vi "TeslaSense Server mimic.vi"() -> ()   [LabVIEW 2019]
doc: "Demonstrates how to set up a basic TCP connection, send data to the specified port once a connection has been established, and terminate the connection once the data has been sent. This VI is designed to stop if the TCP connection is terminated. The data sent in this example is an array of random numbers."
panel:
  in  "Client Closed":string="The client VI closed the connection."
  in  "Stop":bool
  out "data read from client gui (timestamp, thresholds)":string
  out "Array of data read from GUI":dbl[](array[numeric])
  out "Timestamp":dbl
  out "appended array":dbl[](array[numeric])
  out "length":i32
  # "This program mimics the TeslaSense server so that the Client can be tested without the launchpad."
  # "1. Make sure bytes read on TeslaSense client is 82"
  # "2. Make sure TeslaSense client opens connection with 'localhost'"
  # "3. Start client first"
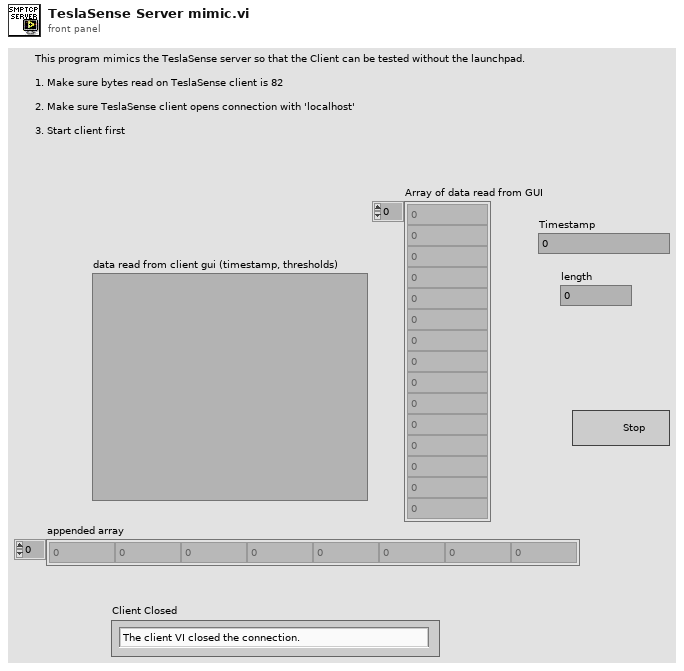
[diagram p1: front panel]
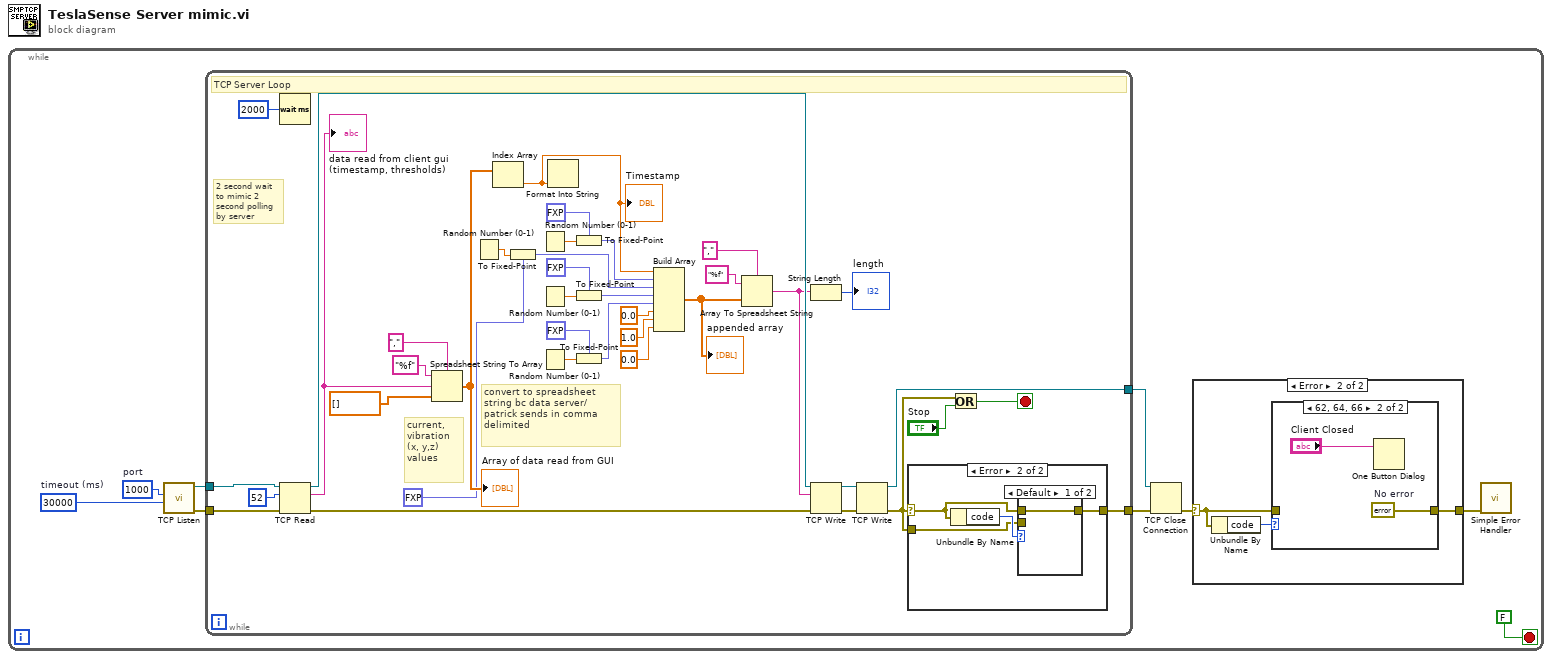
[diagram p0: block diagram]
diagram:
  n1 = while {
    stop <- FALSE stop-if-true
    w4 = u16 1000  # port
    w5 = 30000  # timeout (ms)
    n2 = call <vilib>:"TCP Listen.vi"("timeout ms (wait forever: -1)"=w5, "port"=w4) -> ("error out"=w6:errorcluster, "connection ID"=w7:refnum<k5>)  [unwired: 5 in, 3 out]
    n3 = while {
      tunnel: w7 -> [w38]
      tunnel: w6 -> [w37]
      tunnel: [w42] -> w3
      tunnel: [w41] -> w2
      stop <- w17 stop-if-true
      # "2 second wait to mimic 2 second polling by server"
      # "convert to spreadsheet string bc data server/patrick sends in comma delimited"
      # "current, vibration (x, y,z) values"
      # "TCP Server Loop"
      n4 = Wait (ms)(milliseconds to wait=u32 2000) -> ()  [unwired: 1 out]
      n5 = TCP Read(connection ID=w38, bytes to read=52, error in (no error)=w37) -> (connection ID out=w46:refnum<k5>, data out=w52:string, error out=w45:errorcluster)  [unwired: 2 in]
      "data read from client gui (timestamp, thresholds)" <- w52
      n6 = Spreadsheet String To Array(delimiter (Tab)=",", format string="%f", spreadsheet string=w52, array type (2D Dbl)=dbl[] []) -> (array=w51:dbl[])
      "Array of data read from GUI" <- w51
      n7 = Random Number (0-1)() -> (number: 0 to 1=w29:dbl)
      n8 = Index Array(array=w51) -> (element=w50:dbl)  [unwired: 1 in]
      "Timestamp" <- w50
      n9 = To Fixed-Point(fixed-point type=fxp<+/-,32,16> 10.0, number=w29) -> (fixed-point=w28:fxp<+/-,32,16>)
      n10 = Random Number (0-1)() -> (number: 0 to 1=w32:dbl)
      n11 = Random Number (0-1)() -> (number: 0 to 1=w25:dbl)
      n12 = Random Number (0-1)() -> (number: 0 to 1=w23:dbl)
      n13 = Format Into String(w50) -> ()  [unwired: 3 in, 2 out]
      n14 = To Fixed-Point(fixed-point type=fxp<+/-,32,16> 10.0, number=w32) -> (fixed-point=w31:fxp<+/-,32,16>)
      n15 = To Fixed-Point(fixed-point type=fxp<+/-,32,16> 10.0, number=w25) -> (fixed-point=w26:fxp<+/-,32,16>)
      n16 = To Fixed-Point(fixed-point type=fxp<+/-,32,16> 10.0, number=w23) -> (fixed-point=w22:fxp<+/-,32,16>)
      n17 = Build Array(w50, w31, w28, w26, w22, 0.0 ("element"), 1.0 ("element"), 0.0 ("element")) -> (w49:dbl[])
      "appended array" <- w49
      n18 = Array To Spreadsheet String(delimiter (Tab)=",", array=w49, 3:"%f" ("format string")) -> (spreadsheet string=w21:string)
      n19 = String Length(string=w21) -> (length=→"length":i32)
      n20 = TCP Write(connection ID=w46, data in=w21, error in (no error)=w45) -> (connection ID out=w44:refnum<k5>, error out=w43:errorcluster)  [unwired: 2 out]
      n21 = TCP Write(connection ID=w44, error in (no error)=w43) -> (connection ID out=w41:refnum<k5>, error out=w18:errorcluster)  [unwired: 2 in, 1 out]
      n22 = case shown="Error" w18 {
        selector: w18 -> [w56 w59]
        tunnel: [w56 w57] -> w42
        tunnel: w18 -> [_ w58]
        frame No Error {
        }
        frame Error {
          n23 = Unbundle By Name(w59) -> ("code"=w60:i32)
          n24 = case shown="Default" w60 {
            tunnel: w59 -> [w61 _]
            tunnel: w58 -> [_ w62]
            tunnel: [w61 w62] -> w57
            frame Default {
            }
            frame 56 {
            }
          }
        }
      }
      n25 = Or(x=w18, y="Stop") -> (x .or. y?=w17:bool)
    }
    n26 = TCP Close Connection(connection ID=w2, error in (no error)=w3) -> (error out=w9:errorcluster)  [unwired: 2 out]
    n27 = case shown="Error" w9 {
      selector: w9 -> [w10 w12]
      tunnel: [w10 w11] -> w8
      frame No Error {
      }
      frame Error {
        n28 = Unbundle By Name(w12) -> ("code"=w13:i32)
        n29 = case shown="62, 64, 66" w13 {
          tunnel: w12 -> [w14 _]
          tunnel: [w14 w16] -> w11
          frame Default {
          }
          frame 62, 64, 66 {
            w16 = errorcluster {"status"=FALSE, "code"=0, "source"=""}  # No error
            n30 = One Button Dialog(message="Client Closed") -> ()  [unwired: 1 in, 1 out]
          }
        }
      }
    }
    n31 = call <vilib>:"Simple Error Handler.vi"("error in (no error)"=w8) -> ()  [unwired: 1 in, 8 out]
  }
